vi "Hold.vi"(8 "error in (no error)":errorcluster, 11 "VISA resource name":refnum<visa-resource-name>) -> (0 "error out":errorcluster, 3 "VISA resource name out":refnum<visa-resource-name>)   [LabVIEW 2014, in "Fluke 190 Series II.lvlib"]
doc: "Sets the Scopemeter in the Hold mode. In more detail: the Scopemeter stops sampling the input channels and stops calculating new measurement results. Bringing the instrument to Hold-mode makes it \"freeze\" the display."
uses:
  Fluke 190 Series II.lvlib
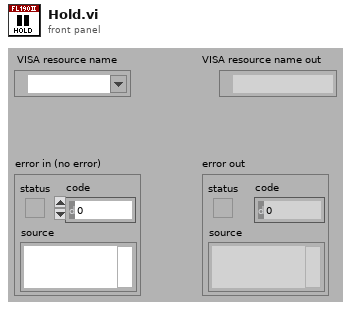
[diagram p1: front panel]
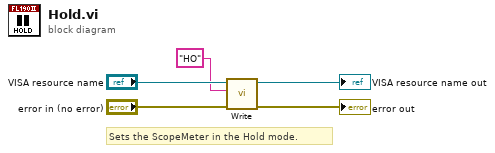
[diagram p0: block diagram]
diagram:
  # "Sets the ScopeMeter in the Hold mode."
  n1 = call "Write.vi"("error in (no error)"="error in (no error)", "Write Buffer"="HO", "VISA resource name"="VISA resource name") -> ("error out"=→"error out":errorcluster, "VISA resource name out"=→"VISA resource name out":refnum<visa-resource-name>)  [unwired: 7 out]
